vi "Float_To_Integer.vi"(10 "Double":dbl) -> (2 "32bit integer":i32)   [LabVIEW 2010]
doc: "Converts a hexadecimal string to a floating-point number (32-bit or 64-bit)\naccording to the IEEE 754 standard. The VI has three inputs: HEX Displayed String, which is the hexadecimal string, 32bit?, which determines if it is computing a single-precision or double-precision floating-point number, and error in, which passes in an error cluster."
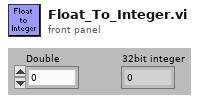
[diagram p1: front panel]
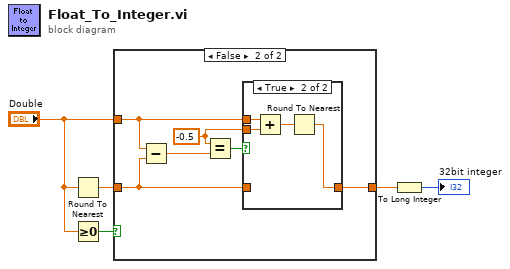
[diagram p0: block diagram]
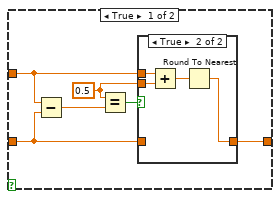
[diagram p2: hidden frame]
diagram:
  n1 = Round To Nearest(number="Double") -> (nearest integer value=w5:dbl)
  n2 = Greater Or Equal To 0?(x="Double") -> (x >= 0?=w4:bool)
  n3 = case shown="False" w4 {
    tunnel: w5 -> [w8 w19]
    tunnel: "Double" -> [w7 w18]
    tunnel: [w6 w17] -> w3
    frame True {
      w9 = 0.5 ("y")
      n4 = Subtract(x=w7, y=w8) -> (x-y=w11:dbl)
      n5 = Equal?(x=w9, y=w11) -> (x = y?=w10:bool)
      n6 = case shown="True" w10 {
        tunnel: w7 -> [_ w16]
        tunnel: w9 -> [_ w15]
        tunnel: w8 -> [w12 _]
        tunnel: [w12 w13] -> w6
        frame False {
        }
        frame True {
          n7 = Add(x=w16, y=w15) -> (x+y=w14:dbl)
          n8 = Round To Nearest(number=w14) -> (nearest integer value=w13:dbl)
        }
      }
    }
    frame False {
      w20 = -0.5 ("y")
      n9 = Subtract(x=w18, y=w19) -> (x-y=w22:dbl)
      n10 = Equal?(x=w20, y=w22) -> (x = y?=w21:bool)
      n11 = case shown="True" w21 {
        tunnel: w18 -> [_ w27]
        tunnel: w20 -> [_ w26]
        tunnel: w19 -> [w23 _]
        tunnel: [w23 w24] -> w17
        frame False {
        }
        frame True {
          n12 = Add(x=w27, y=w26) -> (x+y=w25:dbl)
          n13 = Round To Nearest(number=w25) -> (nearest integer value=w24:dbl)
        }
      }
    }
  }
  n14 = To Long Integer(number=w3) -> (32bit integer=→"32bit integer":i32)
